vi "HotOrCold.vi"(11 "Numeric":dbl) -> (3 "cold":dbl)   [LabVIEW 2015]
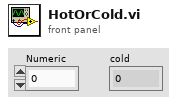
[diagram p1: front panel]
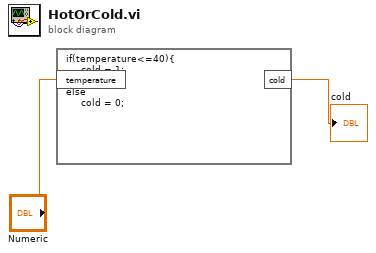
[diagram p0: block diagram]
diagram:
  n1 = formula code="if(temperature<=40){\n     cold = 1;\n}\nelse\n     cold = 0;"("temperature"="Numeric") -> ("cold"=→"cold":dbl)
